vi "VI2.vi"(8 "Numeric":dbl=4.0) -> (0 "Numeric 2":dbl)   [LabVIEW 2023]
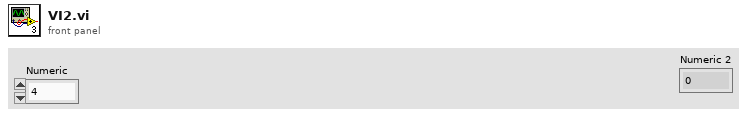
[diagram p1: front panel]
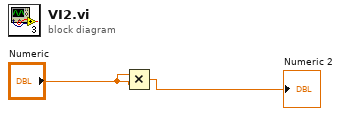
[diagram p0: block diagram]
diagram:
  n1 = Multiply(x="Numeric", y="Numeric") -> (x*y=→"Numeric 2":dbl)
